vi "Set Equalization Mode.vi"(8 "error in":errorcluster, 10 "equalization mode":T1, 11 "eye scan in":refnum<class "niHighSpeedSerial Eye Scan v1 Host.lvclass">) -> (0 "error out":errorcluster, 3 "eye scan out":refnum<class "niHighSpeedSerial Eye Scan v1 Host.lvclass">)   [LabVIEW 2014, in "niHighSpeedSerial Eye Scan v1 Host.lvclass"]
doc: "Sets the Equalization Mode of the receiver. This must match the Equalization Mode that the FPGA is configured to use.\n\n<B>Input Parameters</B>\n\n<B>error in</B> describes error conditions that occur before this node runs. This input provides standard 'error in' functionality.\n\n<B>equalization mode</B> indicates the Equalization Mode that the lane is using.\nenum values: DFE,LPM\n\n<B>eye scan in</B> Takes in a reference to your session from the previous VI.\n\n<B>Output Parameters</B>\n\n<B>error out</B> contains error information. This output provides standard 'error out' functionality.\n\n<B>eye scan out</B> passes a reference to your session to the next VI."
uses:
  <instrlib>/niHighSpeedSerial/Eye Scan/v1/Host/Eye Scan/niHighSpeedSerial Eye Scan v1 Host.lvclass
  <instrlib>/niHighSpeedSerial/Eye Scan/v1/Host/Common/Public/Equalization Mode.ctl
  <instrlib>/niHighSpeedSerial/Eye Scan/v1/Host/Eye Scan/niHighSpeedSerial Eye Scan v1 Host.lvclass/niHighSpeedSerial Eye Scan v1 Host.ctl
  <vilib>/Utility/error.llb/Error Cluster From Error Code.vi
  <vilib>/ErrorRing/Error Ring.xnode
  <instrlib>/niHighSpeedSerial/Eye Scan/v1/Host/Common/niHighSpeedSerial Eye Scan Common v1 Host.lvlib
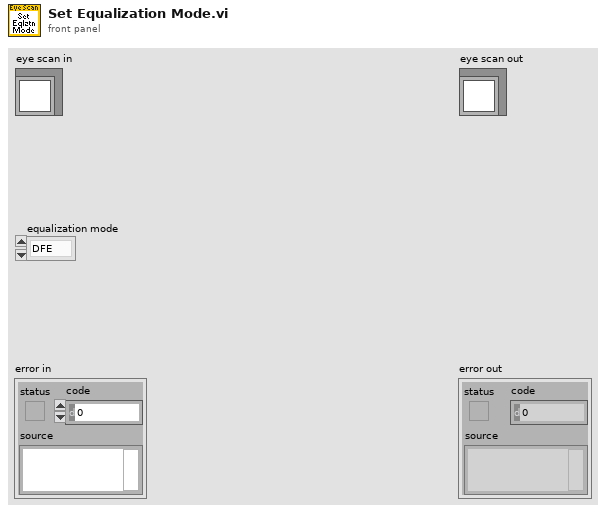
[diagram p1: front panel]
types:
  T1 = typedef "niHighSpeedSerial Eye Scan Common v1 Host.lvlib/Equalization Mode.ctl" = enum16{"DFE", "LPM"}
  T2 = typedef "niHighSpeedSerial Eye Scan v1 Host.lvclass/Private Data.ctl" = cluster{"instruction target":refnum<class "niInstr Instruction Target v1 Host.lvclass">, "channels":T3[], "measure state":T4, "rx output divider":T5, "equalization mode":T1, "rx data width":T6, "BER floor":dbl, "number of points completed":i32, "rx output divider configured?":bool, "equalization mode configured?":bool, "rx data width configured?":bool}
  T3 = typedef "niHighSpeedSerial Eye Scan v1 Host.lvclass/Channel Data.ctl" = cluster{"instance":u8, "channel":refnum<class "niHighSpeedSerial Eye Scan Single Point v1 Host.lvclass">, "point iterator":refnum<class "niHighSpeedSerial Eye Scan Point Iterator v1 Host.lvclass">}
  T4 = typedef "niHighSpeedSerial Eye Scan v1 Host.lvclass/Measure State.ctl" = enum16{"Uninitialized", "Initialized", "Ready", "Measuring", "Finished", "Aborted"}
  T5 = typedef "niHighSpeedSerial Eye Scan Common v1 Host.lvlib/RX Output Divider.ctl" = enum16{"1", "2", "4", "8", "16"}
  T6 = typedef "niHighSpeedSerial Eye Scan Common v1 Host.lvlib/Data Width.ctl" = enum16{"16 Bit", "20 Bit", "32 Bit", "40 Bit"}
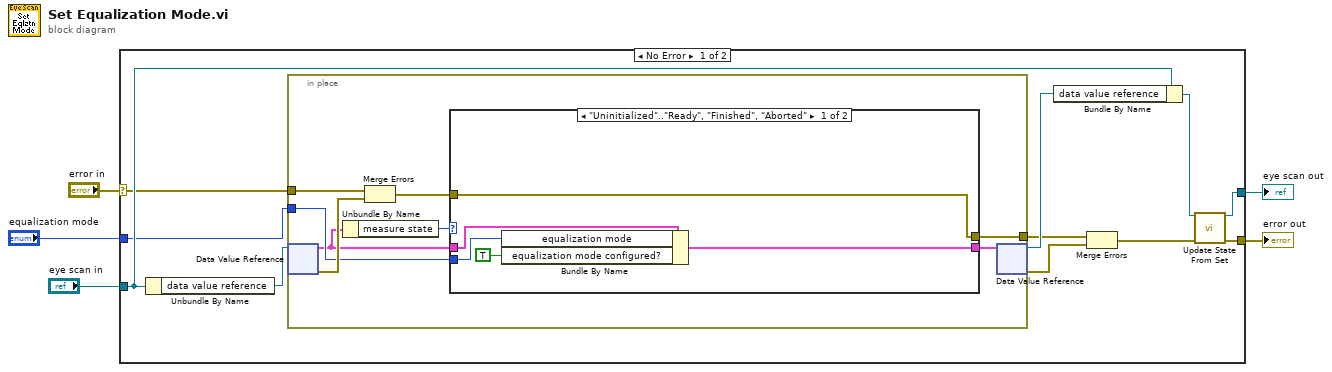
[diagram p0: block diagram]
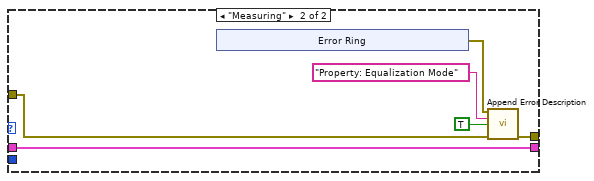
[diagram p2: hidden frame]
diagram:
  n1 = case shown="No Error" "error in" {
    selector: "error in" -> [w10 w41]
    tunnel: [w8 w41] -> w4
    tunnel: [w6 w40] -> w2
    tunnel: "eye scan in" -> [w14 w40]
    tunnel: "equalization mode" -> [w13 _]
    frame No Error {
      n2 = Unbundle By Name(w14) -> ("data value reference"=w16:refnum<data-value>)
      n3 = in-place {
        in-place-border: w13 -> [w22]
        in-place-border: [w19] -> w12
        in-place-border: w10 -> [w24]
        n4 = in-place-dvr #1(w16) -> (w18:T2, w23:errorcluster)
        n5 = Unbundle By Name(w18) -> ("measure state"=w17:T4)
        n6 = Merge Errors(w24, w23) -> (w20:errorcluster)
        n7 = case shown="\"Uninitialized\"..\"Ready\", \"Finished\", \"Aborted\"" w17 {
          tunnel: w20 -> [w29 w33]
          tunnel: [w29 w32] -> w19
          tunnel: w22 -> [w27 _]
          tunnel: w18 -> [w28 w35]
          tunnel: [w26 w35] -> w21
          frame "Uninitialized".."Ready", "Finished", "Aborted" {
            n8 = Bundle By Name(cluster=w28, "equalization mode"=w27, "equalization mode configured?"=TRUE) -> (w26:T2)
          }
          frame "Measuring" {
            n9 = xnode "Error Ring"() -> ("error out"=w34:errorcluster)
            n10 = call <instrlib>:"Append Error Description.vi"("error to append"=w34, "append string (\"\")"="Property: Equalization Mode" ("append string (\"\")"), "generate error?"=TRUE, "error in"=w33) -> ("error out"=w32:errorcluster)  [unwired: 11 in]
          }
        }
        n11 = in-place-dvr #1(w21) -> (w15:refnum<data-value>, w11:errorcluster)
      }
      n12 = Bundle By Name(cluster=w14, "data value reference"=w15) -> (w7:refnum<class "niHighSpeedSerial Eye Scan v1 Host.lvclass">)
      n13 = Merge Errors(w12, w11) -> (w9:errorcluster)
      n14 = call <instrlib>:"Update State From Set.vi"("eye scan in"=w7, "error in"=w9) -> ("eye scan out"=w6:refnum<class "niHighSpeedSerial Eye Scan v1 Host.lvclass">, "error out"=w8:errorcluster)  [unwired: 12 in]
    }
    frame Error {
    }
  }
  "error out" <- w4
  "eye scan out" <- w2
